vi "String to 1D Array 2.vi"(7 "delimiter (,)":string=",", 8 "Error in":errorcluster caption="Error in (no error)", 10 "string":string) -> (0 "Error out":errorcluster, 1 "Array of Strings":string[](array[string])=["sin(x)+2", "VIA(x", "y)", " VIB(z)"])   [LabVIEW 2017, in "API String Arguments Support.lvlib"]
uses:
  API String Arguments Support.lvlib
  <userlib>/_NEVSTOP/Communicable State Machine(CSM)/Communicable State Machine.lvlib
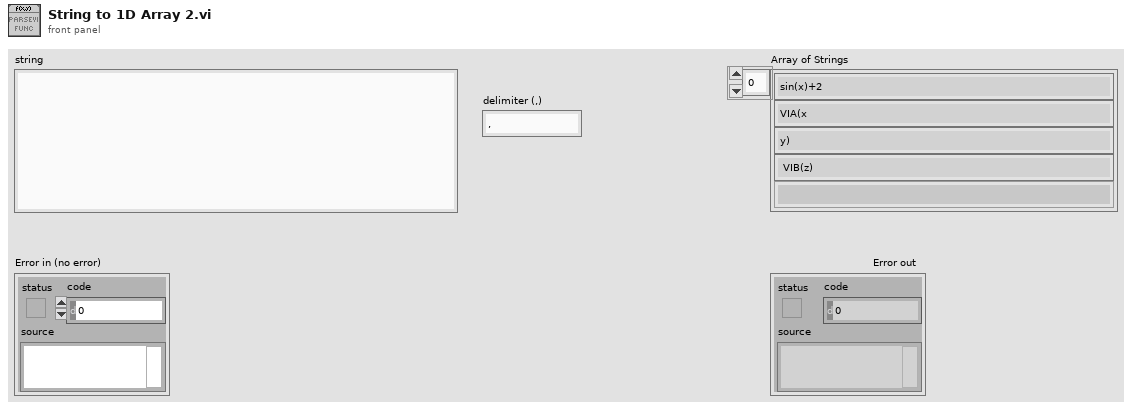
[diagram p1: front panel]
types:
  T1 = enum16{"0x2829 - ()", "0x5B5D - []", "0x7B7D - {}"}
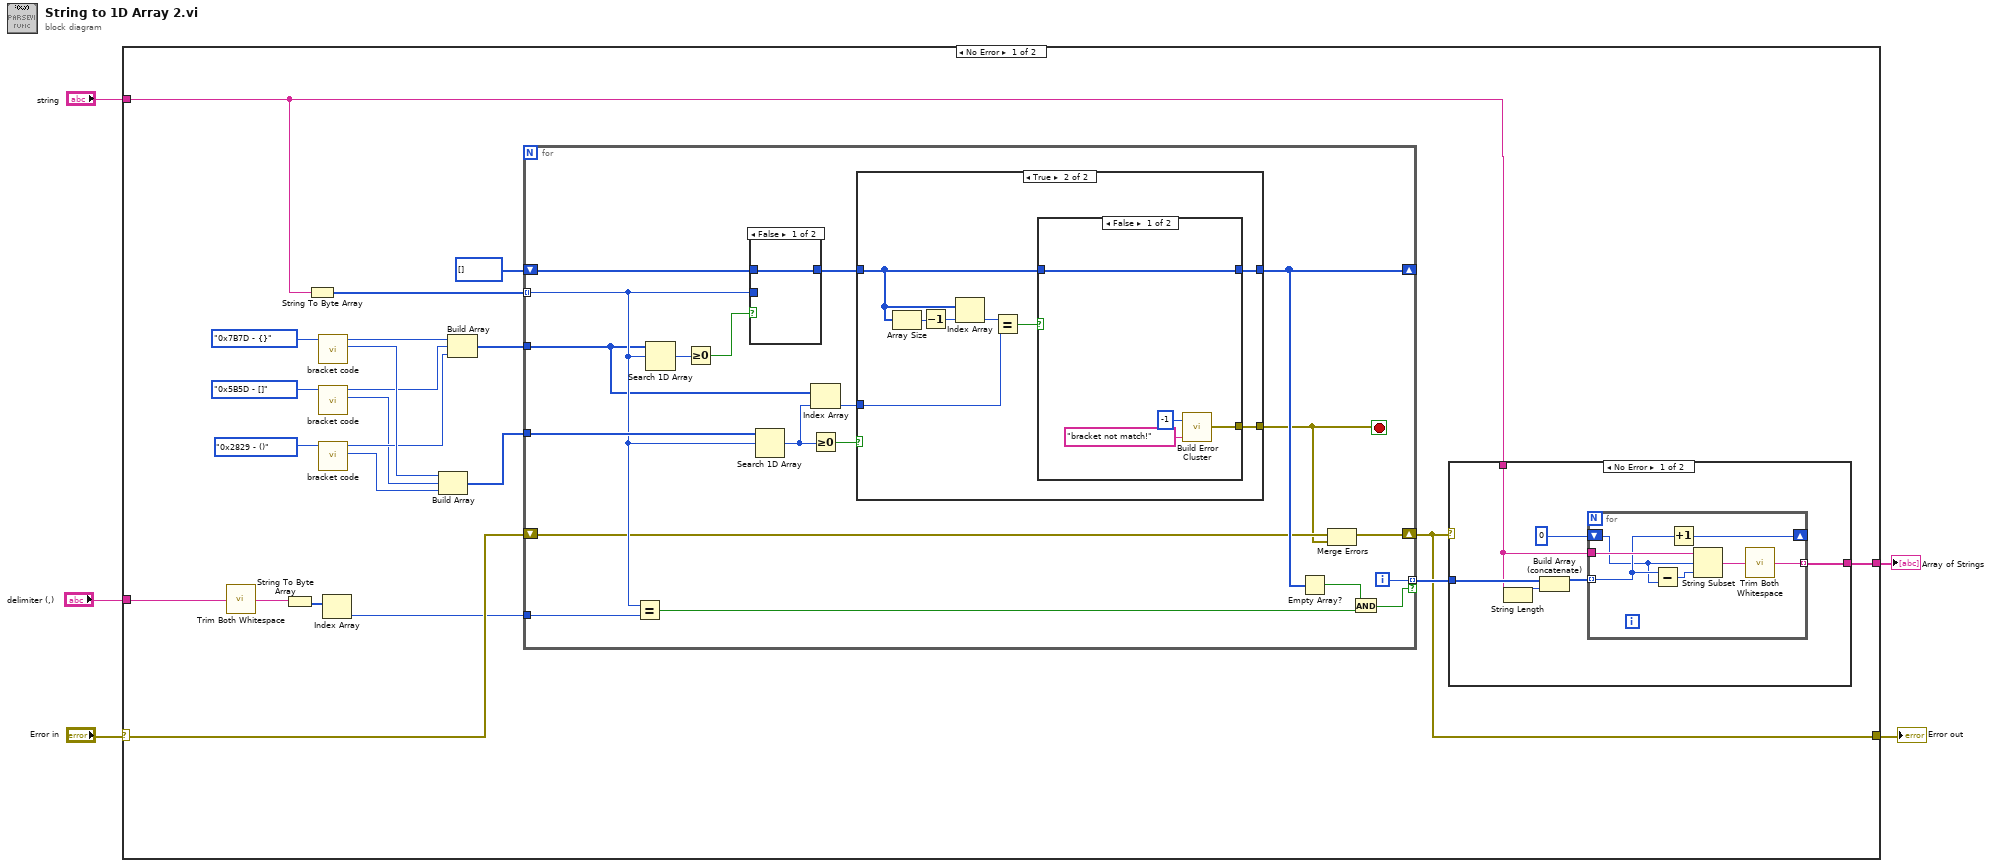
[diagram p0: block diagram]
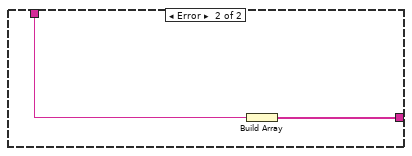
[diagram p2: hidden frame]
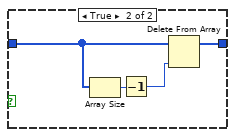
[diagram p4: hidden frame]
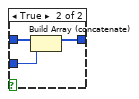
[diagram p5: hidden frame]
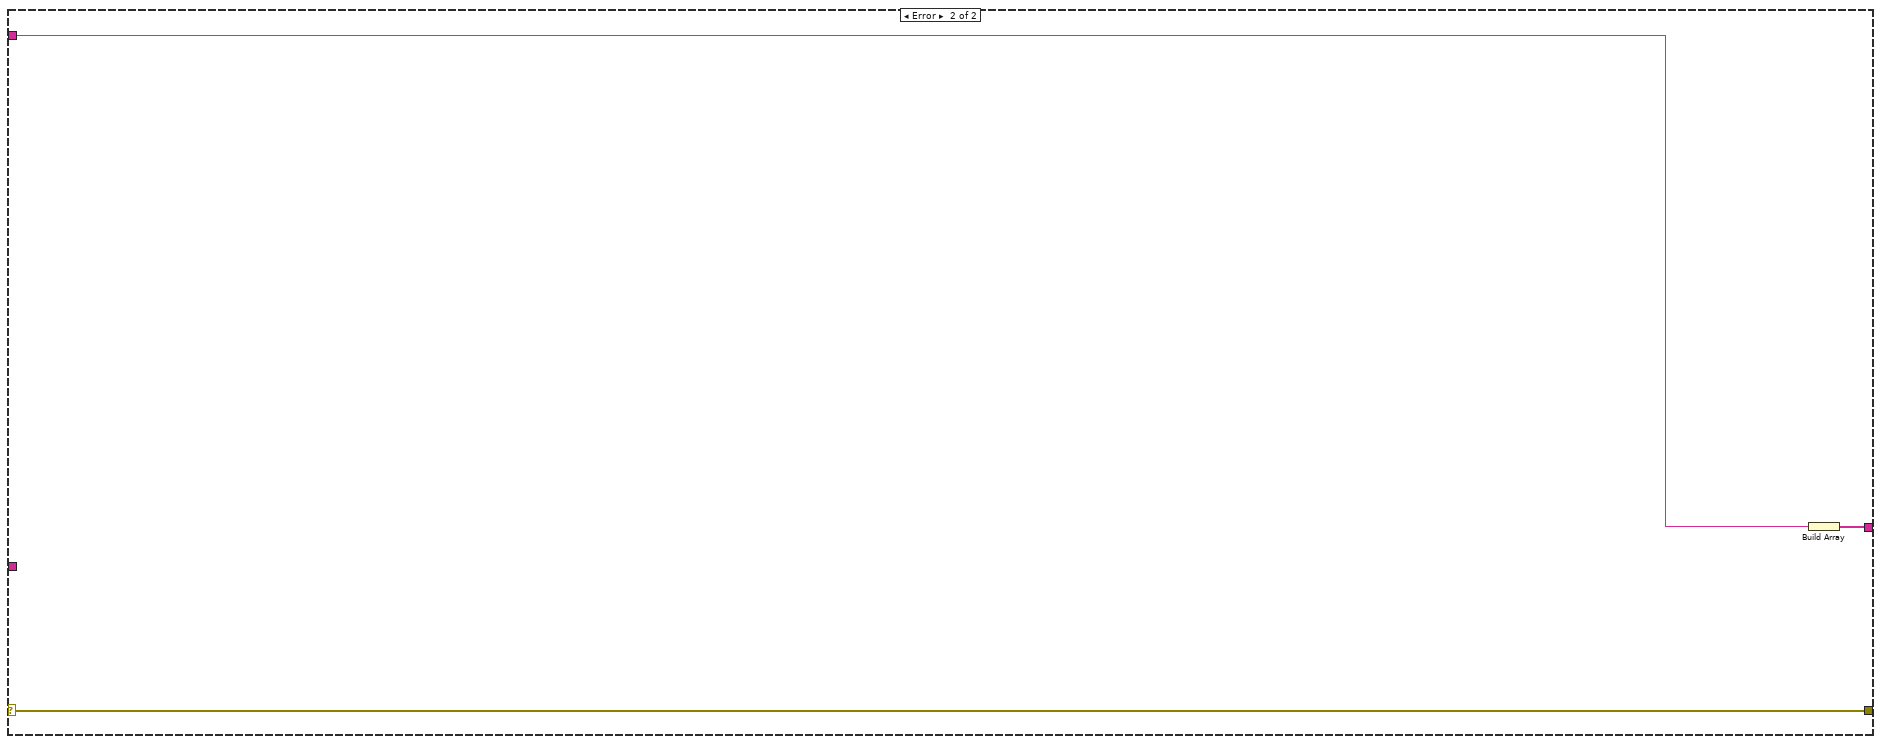
[diagram p6: hidden frame]
diagram:
  n1 = case shown="No Error" "Error in" {
    selector: "Error in" -> [w11 w85]
    tunnel: [w24 w84] -> w5
    tunnel: "string" -> [w21 w83]
    tunnel: [w10 w85] -> w2
    tunnel: "delimiter (,)" -> [w9 _]
    frame No Error {
      n2 = call <userlib>:"Trim Both Whitespace.vi"("string"=w9) -> ("trimmed string"=w6:string)  [unwired: 1 in]
      n3 = String To Byte Array(string=w6) -> (unsigned byte array=w8:u8[])
      n4 = String To Byte Array(string=w21) -> (unsigned byte array=w26:u8[])
      n5 = call "bracket code.vi"("Enum"=T1."0x7B7D - {}" ("TYPE")) -> ("Numeric"=w17:u8, "Numeric 2"=w22:u8)  [unwired: 9 in]
      n6 = call "bracket code.vi"("Enum"=T1."0x5B5D - []" ("TYPE")) -> ("Numeric"=w14:u8, "Numeric 2"=w16:u8)  [unwired: 9 in]
      n7 = call "bracket code.vi"("Enum"=T1."0x2829 - ()" ("TYPE")) -> ("Numeric"=w13:u8, "Numeric 2"=w15:u8)  [unwired: 9 in]
      n8 = Index Array(array=w8) -> (element=w7:u8)  [unwired: 1 in]
      n9 = Build Array(w17, w14, w13) -> (w12:u8[])
      n10 = Build Array(w22, w16, w15) -> (w18:u8[])
      n11 = for {
        tunnel: w26 -> [w49] mode=indexing
        shift-right: [w57] -> _
        shift-left: u8[] [] -> [w60]
        tunnel: [w59] -> w25 mode=indexing if=w56
        tunnel: w18 -> [w44]
        tunnel: w12 -> [w51]
        tunnel: w7 -> [w54]
        shift-right: [w47] -> w10
        shift-left: w11 -> [w48]
        i -> [w59]
        stop <- w46 stop-if-true
        n12 = Equal?(x=w49, y=w54) -> (x = y?=w55:bool)
        n13 = Search 1D Array(1D array=w44, element=w49) -> (index of element=w53:i32)  [unwired: 1 in]
        n14 = Greater Or Equal To 0?(x=w53) -> (x >= 0?=w52:bool)
        n15 = case shown="False" w52 {
          tunnel: w60 -> [w79 w82]
          tunnel: w49 -> [_ w81]
          tunnel: [w79 w80] -> w61
          frame False {
          }
          frame True {
            n16 = Build Array (concatenate)(w82, w81) -> (w80:u8[])
          }
        }
        n17 = Search 1D Array(1D array=w51, element=w49) -> (index of element=w43:i32)  [unwired: 1 in]
        n18 = Index Array(array=w44, index=w43) -> (element=w45:u8)
        n19 = Greater Or Equal To 0?(x=w43) -> (x >= 0?=w50:bool)
        n20 = case shown="True" w50 {
          tunnel: w61 -> [w62 w67]
          tunnel: [w62 w70] -> w57
          tunnel: w45 -> [_ w65]
          tunnel: [_ w63] -> w46
          frame False {
          }
          frame True {
            n21 = Array Size(array=w67) -> (size(s)=w69:i32)
            n22 = Decrement(x=w69) -> (x-1=w68:i32)
            n23 = Index Array(array=w67, index=w68) -> (element=w66:u8)
            n24 = Equal?(x=w66, y=w65) -> (x = y?=w64:bool)
            n25 = case shown="False" w64 {
              tunnel: w67 -> [w74 w77]
              tunnel: [w74 w75] -> w70
              tunnel: [w71 _] -> w63
              frame False {
                n26 = call <userlib>:"Build Error Cluster.vi"("String to Prepend to source (\"\")"="bracket not match!" ("String to Prepend to source (\"\")"), "code"=-1) -> ("error out"=w71:errorcluster)
              }
              frame True {
                n27 = Array Size(array=w77) -> (size(s)=w78:i32)
                n28 = Decrement(x=w78) -> (x-1=w76:i32)
                n29 = Delete From Array(array=w77, index=w76) -> (array with subset deleted=w75:u8[])  [unwired: 1 in, 1 out]
              }
            }
          }
        }
        n30 = Empty Array?(array=w57) -> (empty?=w58:bool)
        n31 = Merge Errors(w48, w46) -> (w47:errorcluster)
        n32 = And(x=w58, y=w55) -> (x .and. y?=w56:bool)
      }
      n33 = case shown="No Error" w10 {
        tunnel: w25 -> [w33 _]
        tunnel: [w31 w41] -> w24
        tunnel: w21 -> [w28 w42]
        frame No Error {
          n34 = String Length(string=w28) -> (length=w29:i32)
          n35 = Build Array (concatenate)(w33, w29) -> (w30:i32[])
          n36 = for {
            tunnel: w28 -> [w40]
            tunnel: w30 -> [w38] mode=indexing
            tunnel: [w34] -> w31 mode=indexing
            shift-right: [w35] -> _
            shift-left: 0 ("Numeric") -> [w36]
            n37 = Subtract(x=w38, y=w36) -> (x-y=w37:i32)
            n38 = Increment(x=w38) -> (x+1=w35:i32)
            n39 = String Subset(string=w40, offset (0)=w36, length (rest)=w37) -> (substring=w39:string)
            n40 = call <userlib>:"Trim Both Whitespace.vi"("string"=w39) -> ("trimmed string"=w34:string)  [unwired: 1 in]
          }
        }
        frame Error {
          n41 = Build Array(w42) -> (w41:string[])
        }
      }
    }
    frame Error {
      n42 = Build Array(w83) -> (w84:string[])
    }
  }
  "Array of Strings" <- w5
  "Error out" <- w2
